vi "Bamocar Main.vi"(8 "Error In":errorcluster, 9 "Value to Write":string="3D0059X", 10 "Register":string="3D0059X", 11 "Command":enum16{"Write/Read", "Write", "Read"}(ring)) -> (3 "Decimal":u32)   [LabVIEW 2017]
panel:
  in  "Enum":enum16{""}(ring)
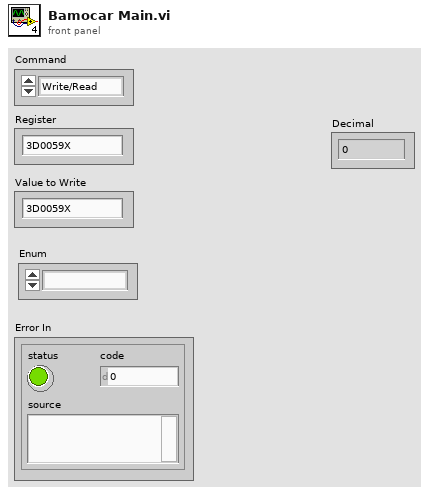
[diagram p1: front panel]
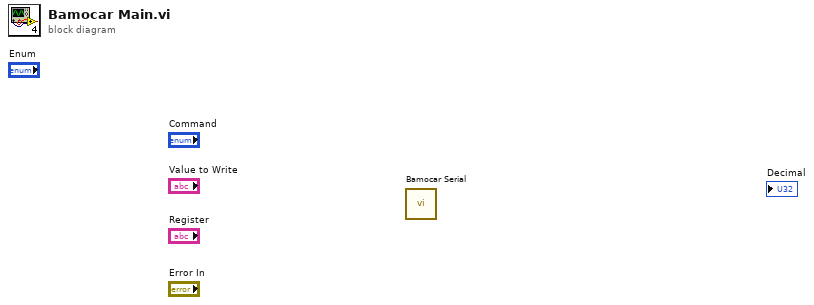
[diagram p0: block diagram]
diagram:
  n1 = call "Bamocar Serial.vi"() -> ()  [unwired: 10 in, 2 out]
